vi "ZMQTestPublisher.vi"() -> ()   [LabVIEW 2017]
uses:
  <vilib>/addons/zeromq/socket_type.ctl
  <vilib>/Platform/TimedLoop/XDataNode/timing_clust.ctl
  <vilib>/Platform/TimedLoop/XDataNode/nitl_modes.ctl
  <vilib>/Platform/TimedLoop/XDataNode/wakeup.ctl
  <vilib>/addons/zeromq/zmq_socket.lvclass
  <vilib>/platform/TimedLoop/XDataNode/XDataNode.xnode
  <vilib>/addons/zeromq/zmq_context.lvclass
  <vilib>/addons/zeromq/zeromq.lvlib
  <vilib>/Platform/TimedLoop/XDataNode/XDNodeRunTimeDep.lvlib
panel:
  out "error out":errorcluster
  in  "Send long event?":bool
  in  "Send short event?":bool
  in  "port":u16=5560
  in  "Stop Button":bool
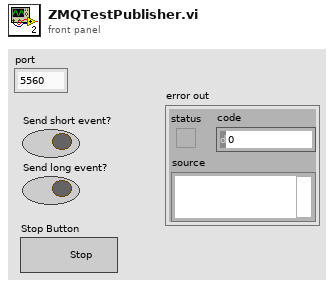
[diagram p1: front panel]
types:
  T1 = typedef "zeromq.lvlib/socket_type.ctl" = enum8{"ZMQ_PAIR", "ZMQ_PUB", "ZMQ_SUB", "ZMQ_REQ", "ZMQ_REP", "ZMQ_DEALER", "ZMQ_ROUTER", "ZMQ_PULL", "ZMQ_PUSH", "ZMQ_XPUB", "ZMQ_XSUB"}
  T2 = typedef "XDNodeRunTimeDep.lvlib/timing_clust.ctl" = cluster{"Expected End [f-1]":u64, "Actual End [f-1]":u64, "Finished Late? [f-1]":bool, "Expected End [i-1]":u64, "Actual End [i-1]":u64, "Finished Late? [i-1]":bool, "Expected Start [i]":u64, "Actual Start [i]":u64, "Expected Start [f]":u64, "Actual Start [f]":u64, "Source Name":string, "Structure Name":string, "Period":i64, "Deadline":i64, "Offset":i64, "Start":i64, "Priority":i32, "Timeout":i32, "Mode":T3, "Wakeup Reason":T4, "Error":errorcluster, "Source Type":string, "Secondary Source Type":string, "Global End Time":u64, "Global Start Time":u64, "Frame Duration":u64, "Iteration Duration":u64, "Assigned CPU":i32, "I/O Scan Engine Mode":u32}
  T3 = typedef "XDNodeRunTimeDep.lvlib/nitl_modes.ctl" = enum32{"No Change", "Process missed periods, maintain original phase", "Discard missed periods, maintain original phase", "Process missed periods, ignore original phase", "Discard missed periods, ignore original phase"}
  T4 = typedef "XDNodeRunTimeDep.lvlib/wakeup.ctl" = enum32{"Normal", "Aborted", "Asynchronous wakeup", "Timing source error", "Timed loop error", "Timeout"}
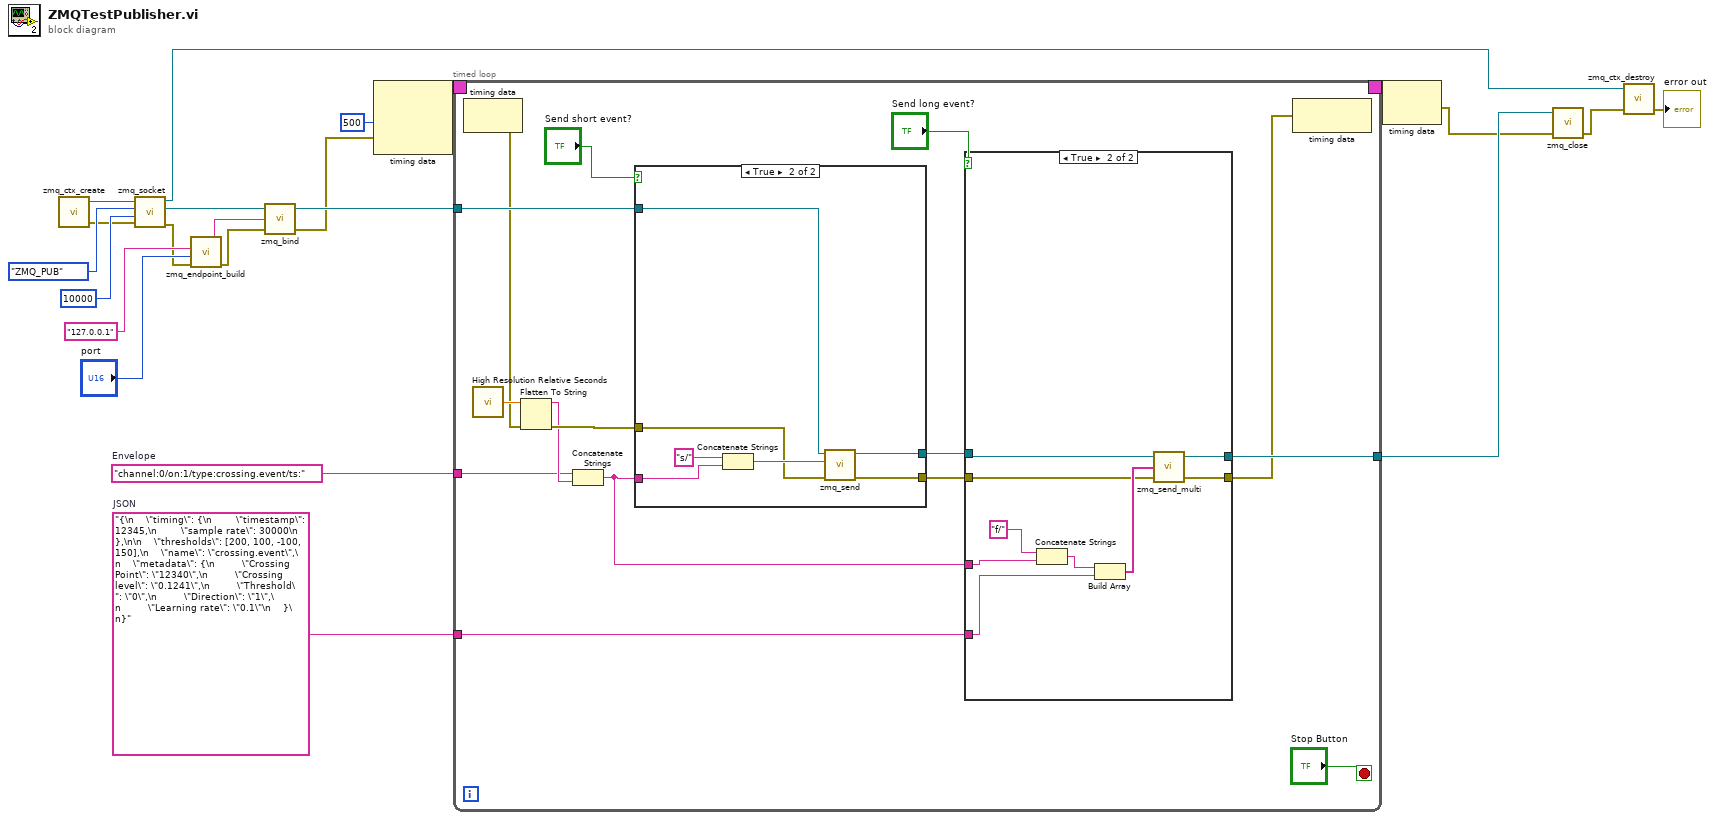
[diagram p0: block diagram]
diagram:
  w6 = "{\n    \"timing\": {\n        \"timestamp\": 12345,\n        \"sample rate\": 30000\n    },\n\n    \"thresholds\": [200, 100, -100, 150],\n    \"name\": \"crossing.event\",\n    \"metadata\": {\n         \"Crossing Point\": \"12340\",\n         \"Crossing level\": \"0.1241\",\n         \"Threshold\": \"0\",\n         \"Direction\": \"1\",\n         \"Learning rate\": \"0.1\"\n    }\n}"  # JSON
  w5 = "channel:0/on:1/type:crossing.event/ts:"  # Envelope
  n1 = call <vilib>:"zmq_ctx_create.vi"() -> ("error out"=w18:errorcluster, "context out"=w21:refnum<class "zmq_context.lvclass">)  [unwired: 4 in]
  n2 = call <vilib>:"zmq_socket.vi"("error in"=w18, "linger (ms)"=10000, "socket type"=socket_type."ZMQ_PUB", "context in"=w21) -> ("error out"=w14:errorcluster, "socket out"=w17:refnum<class "zmq_socket.lvclass">, "context out"=w22:refnum<class "zmq_context.lvclass">)  [unwired: 1 in]
  n3 = call <vilib>:"zmq_endpoint_build.vi"("error in"=w14, "port"="port", "address"="127.0.0.1" ("initial string")) -> ("error out"=w13:errorcluster, "endpoint"=w12:string)  [unwired: 2 in, 1 out]
  n4 = call <vilib>:"zmq_bind.vi"("error in"=w13, "endpoint"=w12, "socket in"=w17) -> ("error out"=w7:errorcluster, "socket out"=w11:refnum<class "zmq_socket.lvclass">)  [unwired: 1 in]
  n5 = node-c288(i64 500 ("Period"), w7) -> (w10:T2)  [unwired: 1 in]
  n6 = timed-loop {
    tunnel: w11 -> [w36]
    timing: w10 -> [_]
    timing-out: [_] -> w9
    tunnel: w6 -> [w26]
    tunnel: w5 -> [w29]
    tunnel: [w24] -> w4
    stop <- "Stop Button" stop-if-true
    n7 = node-c288() -> (w32:errorcluster)  [unwired: 1 in]
    n8 = call <vilib>:"High Resolution Relative Seconds.vi"() -> ("relative seconds"=w33:dbl)
    n9 = Flatten To String(anything=w33, error in (no error)=w32) -> (data string=w30:string, error out=w31:errorcluster)  [unwired: 2 in, 1 out]
    n10 = Concatenate Strings(w29, w30) -> (w25:string)
    n11 = case "Send short event?" shown="True" "Send short event?" {
      tunnel: w36 -> [w49 w54]
      tunnel: w31 -> [w50 w55]
      tunnel: w25 -> [_ w51]
      tunnel: [w50 w53] -> w28
      tunnel: [w49 w52] -> w27
      frame False {
      }
      frame True {
        n12 = Concatenate Strings("s/" ("string"), w51) -> (w56:string)
        n13 = call <vilib>:"zmq_send.vi"("error in"=w55, "data"=w56, "socket in"=w54) -> ("error out"=w53:errorcluster, "socket out"=w52:refnum<class "zmq_socket.lvclass">)  [unwired: 4 in]
      }
    }
    n14 = case shown="True" "Send long event?" {
      tunnel: w28 -> [w38 w43]
      tunnel: w27 -> [w39 w42]
      tunnel: w26 -> [_ w45]
      tunnel: w25 -> [_ w47]
      tunnel: [w38 w41] -> w23
      tunnel: [w39 w40] -> w24
      frame False {
      }
      frame True {
        n15 = Concatenate Strings("f/" ("string"), w47) -> (w46:string)
        n16 = Build Array(w46, w45) -> (w44:string[])
        n17 = call <vilib>:"zmq_send_multi.vi"("error in"=w43, "parts"=w44, "socket in"=w42) -> ("error out"=w41:errorcluster, "socket out"=w40:refnum<class "zmq_socket.lvclass">)  [unwired: 1 in]
      }
    }
    n18 = node-c288(w23) -> ()  [unwired: 1 out]
  }
  n19 = node-c288(w9) -> (w3:errorcluster)
  n20 = call <vilib>:"zmq_close.vi"("error in"=w3, "socket"=w4) -> ("error out"=w2:errorcluster)  [unwired: 3 in]
  n21 = call <vilib>:"zmq_ctx_destroy.vi"("error in"=w2, "context in"=w22) -> ("error out"=→"error out":errorcluster)  [unwired: 3 in]
